vi "LHF.DB.Mongo.Daemon.Start.vi"(6 "Port (27017)":u32=27017, 8 "error in (no error)":errorcluster, 9 "data folder":path=path "C:/data/db", 10 "mongod path":path=path "C:/Program Files/MongoDB/Server/3.2/bin/mongod.exe", 11 "LHF.DB.Mongo in":refnum<class "LHF.DB.Mongo.lvclass">) -> (0 "error out":errorcluster, 3 "LHF.DB.Mongo out":refnum<class "LHF.DB.Mongo.lvclass">)   [LabVIEW 2013, in "LHF.DB.Mongo.lvclass"]
doc: "Starts daemon in background. Data dir is created automatically if non existent."
uses:
  LHF.DB.Mongo.lvclass
  LHF.DB.Mongo.lvclass/LHF.DB.Mongo.ctl
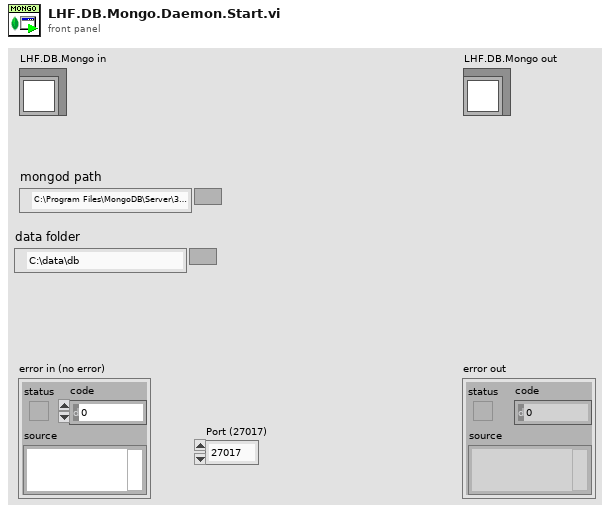
[diagram p1: front panel]
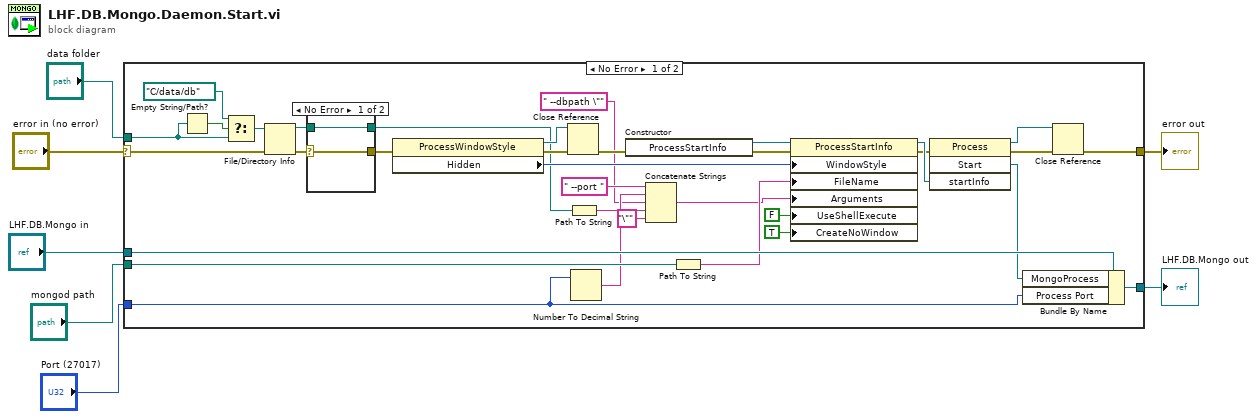
[diagram p0: block diagram]
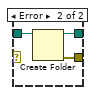
[diagram p2: hidden frame]
diagram:
  n1 = case shown="No Error" "error in (no error)" {
    selector: "error in (no error)" -> [w14 w48]
    tunnel: [w27 w48] -> w6
    tunnel: [w26 w47] -> w4
    tunnel: "LHF.DB.Mongo in" -> [w41 w47]
    tunnel: "mongod path" -> [w40 _]
    tunnel: "data folder" -> [w11 _]
    tunnel: "Port (27017)" -> [w21 _]
    frame No Error {
      n2 = Empty String/Path?(string/path=w11) -> (empty?=w12:bool)
      n3 = Select(t=path "C:/data/db", s=w12, f=w11) -> (s? t:f=w10:path)
      n4 = File/Directory Info(path=w10, error in=w14) -> (path out=w17:path, error out=w18:errorcluster)  [unwired: 5 out]
      n5 = case shown="No Error" w18 {
        selector: w18 -> [w42 _]
        tunnel: w17 -> [w43 w46]
        tunnel: [w43 w45] -> w16
        tunnel: [w42 w44] -> w15
        frame No Error {
        }
        frame Error {
          n6 = Create Folder(path (use dialog)=w46) -> (created path=w45:path, error out=w44:errorcluster)  [unwired: 2 in, 1 out]
        }
      }
      n7 = property class="ProcessWindowStyle"(error in=w15) -> (reference out=w31:refnum<k24>, error out=w32:errorcluster, "Hidden"=w34:i32)  [unwired: 1 in]
      n8 = Close Reference(reference=w31, error in (no error)=w32) -> (error out=w30:errorcluster)
      n9 = Path To String(path=w16) -> (string=w13:string)
      n10 = Number To Decimal String(number=w21) -> (decimal integer string=w22:string)  [unwired: 1 in]
      n11 = constructor class="ProcessStartInfo"(error in=w30) -> (reference out=w38:refnum<k24>, error out=w33:errorcluster)  [unwired: 2 in, 1 out]
      n12 = Concatenate Strings(" --port " ("arguments"), w22, " --dbpath \"" ("arguments"), w13, "\"" ("string")) -> (w19:string)
      n13 = Path To String(path=w40) -> (string=w39:string)
      n14 = property class="ProcessStartInfo"(reference=w38, error in=w33, "WindowStyle"=w34, "FileName"=w39, "Arguments"=w19, "UseShellExecute"=FALSE, "CreateNoWindow"=TRUE) -> (reference out=w36:refnum<k24>, error out=w35:errorcluster)
      n15 = invoke class="Process" method="Start"(error in=w35, "startInfo"=w36) -> (reference out=w28:refnum<k24>, error out=w29:errorcluster, "Start"=w24:refnum<k24>)  [unwired: 2 in, 1 out]
      n16 = Bundle By Name(cluster=w41, "MongoProcess"=w24, "Process Port"=w21) -> (w26:refnum<class "LHF.DB.Mongo.lvclass">)
      n17 = Close Reference(reference=w28, error in (no error)=w29) -> (error out=w27:errorcluster)
    }
    frame Error {
    }
  }
  "error out" <- w6
  "LHF.DB.Mongo out" <- w4
